vi "Read Request Message.vi"(8 "error in (no error)":errorcluster, 11 "Abstract Log Producer in":refnum<class "Abstract Log Producer.lvclass">) -> (0 "error out":errorcluster, 2 "Messaging.lvlib:Abstract Request Message.lvclass":refnum<class "Abstract Request Message.lvclass">, 3 "Abstract Log Producer out":refnum<class "Abstract Log Producer.lvclass">)   [LabVIEW 2020, in "Messaging.lvlib" / "Abstract Log Producer.lvclass"]
uses:
  Abstract Log Producer.lvclass
  Message/Abstract Request Message/Abstract Request Message.lvclass
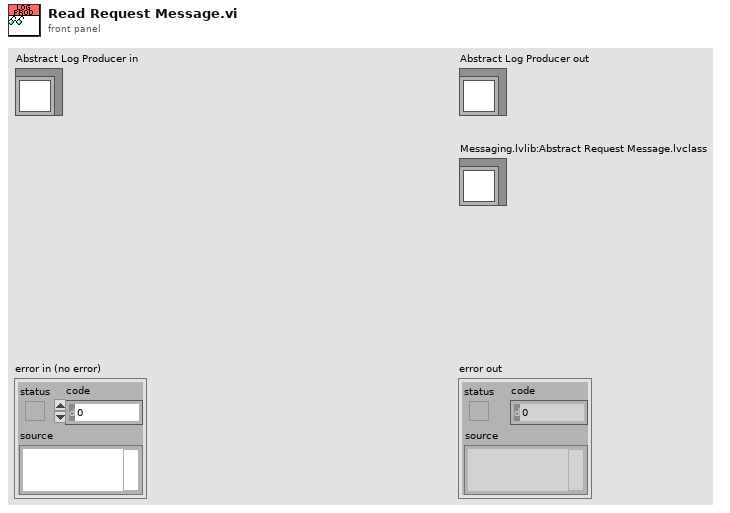
[diagram p1: front panel]
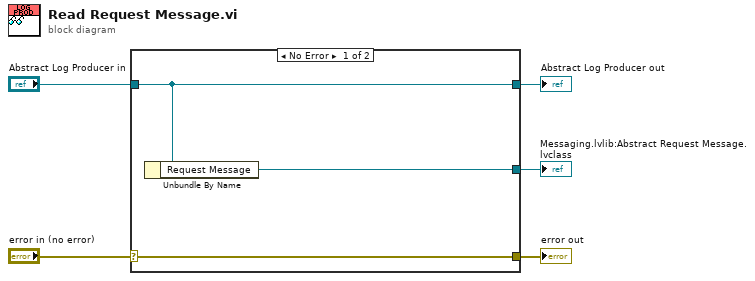
[diagram p0: block diagram]
diagram:
  n1 = case shown="No Error" "error in (no error)" {
    selector: "error in (no error)" -> [w8 w9]
    tunnel: [w8 w9] -> w4
    tunnel: [w7 w10] -> w2
    tunnel: "Abstract Log Producer in" -> [w7 w10]
    tunnel: [w6 _] -> w1
    frame No Error {
      n2 = Unbundle By Name(w7) -> ("Request Message"=w6:refnum<class "Abstract Request Message.lvclass">)
    }
    frame Error {
    }
  }
  "error out" <- w4
  "Abstract Log Producer out" <- w2
  "Messaging.lvlib:Abstract Request Message.lvclass" <- w1
